vi "Close.vi"(8 "error in (no error)":errorcluster, 9 "error in":errorcluster, 10 "Refnum in":T1, 11 "VISA Refnum in":refnum<visa-resource-name>) -> ()   [LabVIEW 2018]
uses:
  <vilib>/addons/database/Connection.llb/Conn ObjectReference.ctl
  <vilib>/addons/database/NI_Database_API.lvlib
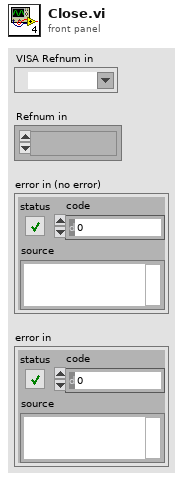
[diagram p1: front panel]
types:
  T1 = typedef "NI_Database_API.lvlib/Conn ObjectReference.ctl" = refnum<k1>
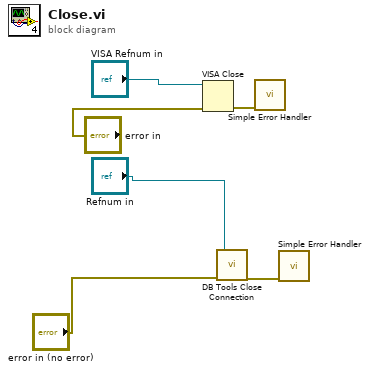
[diagram p0: block diagram]
diagram:
  n1 = VISA Close(VISA resource name="VISA Refnum in", error in (no error)="error in") -> (error out=w3:errorcluster)
  n2 = call <vilib>:"DB Tools Close Connection.vi"("error in (no error)"="error in (no error)", "connection reference"="Refnum in") -> ("error out"=w1:errorcluster)  [unwired: 5 in]
  n3 = call <vilib>:"Simple Error Handler.vi"("error in (no error)"=w3) -> ()  [unwired: 4 in, 5 out]
  n4 = call <vilib>:"Simple Error Handler.vi"("error in (no error)"=w1) -> ()  [unwired: 4 in, 5 out]
